vi "ReadOrSaveCases-UTEX.vi"(9 "Location":enum16{"CUMC", "SERI", "VMR", "Aline", "HSS"}(ring)=enum."SERI", 10 "New Case":T2={"Case Name"="", "Distance between\nscan lines (mm)"=0.0, "Acquistion Parameters"={"Sampling Rate"=0.0, "Ref Delay (ms)"=0.0, "rf points per line"=0, "rf lines"=0, "Dig Scale"=0.0}, "Timeout (s)"=0.0, "Sector?"=FALSE, "Filter Prams"={"low cutoff"=0, "order"=0, "high cutoff"=0}, "Scan Info"={"delay"=0.0, "pivot distance"=0.0, "sector scan angle"=0.0, "operator"="", "Scan Mode"="", "location"=""}, "UT340 Controls"={"High Pass On"=FALSE, "High Pass Filter (MHz)"=1, "Low Pass On"=FALSE, "Low Pass Filter (MHz)"=20, "PE Gain (dB)"=1, "Voltage"=100, "Pulse Width (ns)"=2.0, "Mode"=FALSE, "PC Gain (dB)"=1, "Trig Source"=FALSE, "Rep Rate (Hz)"=0, "PULSE"=FALSE}} {"UT340 Controls"."Low Pass Filter (MHz)" min=20 step=1; "UT340 Controls"."High Pass Filter (MHz)" min=1 max=20 step=1; "UT340 Controls"."Pulse Width (ns)" min=2.0 max=71.75; "UT340 Controls"."Voltage" min=100 max=250 step=2; "UT340 Controls"."PC Gain (dB)" min=0 max=63 step=1; "UT340 Controls"."PE Gain (dB)" min=-6 max=57 step=1}, 11 "Save(T)\\Read(F)":bool) -> (2 "Case List":string[](array[string]), 3 "CaseArray":T3(array[cluster]) {"UT340 Controls"."Low Pass Filter (MHz)" min=20 step=1; "UT340 Controls"."High Pass Filter (MHz)" min=1 max=20 step=1; "UT340 Controls"."Pulse Width (ns)" min=2.0 max=71.75; "UT340 Controls"."Voltage" min=100 max=250 step=2; "UT340 Controls"."PC Gain (dB)" min=0 max=63 step=1; "UT340 Controls"."PE Gain (dB)" min=-6 max=57 step=1})   [LabVIEW 2022 SP3]
uses:
  ScanningControl/Pulsers/UTEX/Controls/UTEX Controls.ctl
  ScanningControl/Digitizers/-DigitizerRoutines/Digitizer.ctl
panel:
  out "path":path
  in  "Acquistion Parameters":T4={"Sampling Rate"=250.0, "Ref Delay (ms)"=0.0, "rf points per line"=2048, "rf lines"=256, "Dig Scale"=4.0} {"Dig Scale" items=["5 V"=5.0, "2 V"=2.0, "1 V"=1.0, "500 mV"=0.5, "200 mV"=0.2, "100 mV"=0.1, "50 mV"=0.05]; "rf lines" min=1; "rf points per line" min=1; "Ref Delay (ms)" format="%.2f"}
  in  "Sector?":bool=TRUE
  in  "Filter Prams":T5={"low cutoff"=20, "order"=81, "high cutoff"=60}
  in  "Timeout (s)":dbl=0.15
  in  "Probe":T6(ring)
  in  "Scan Info":T7
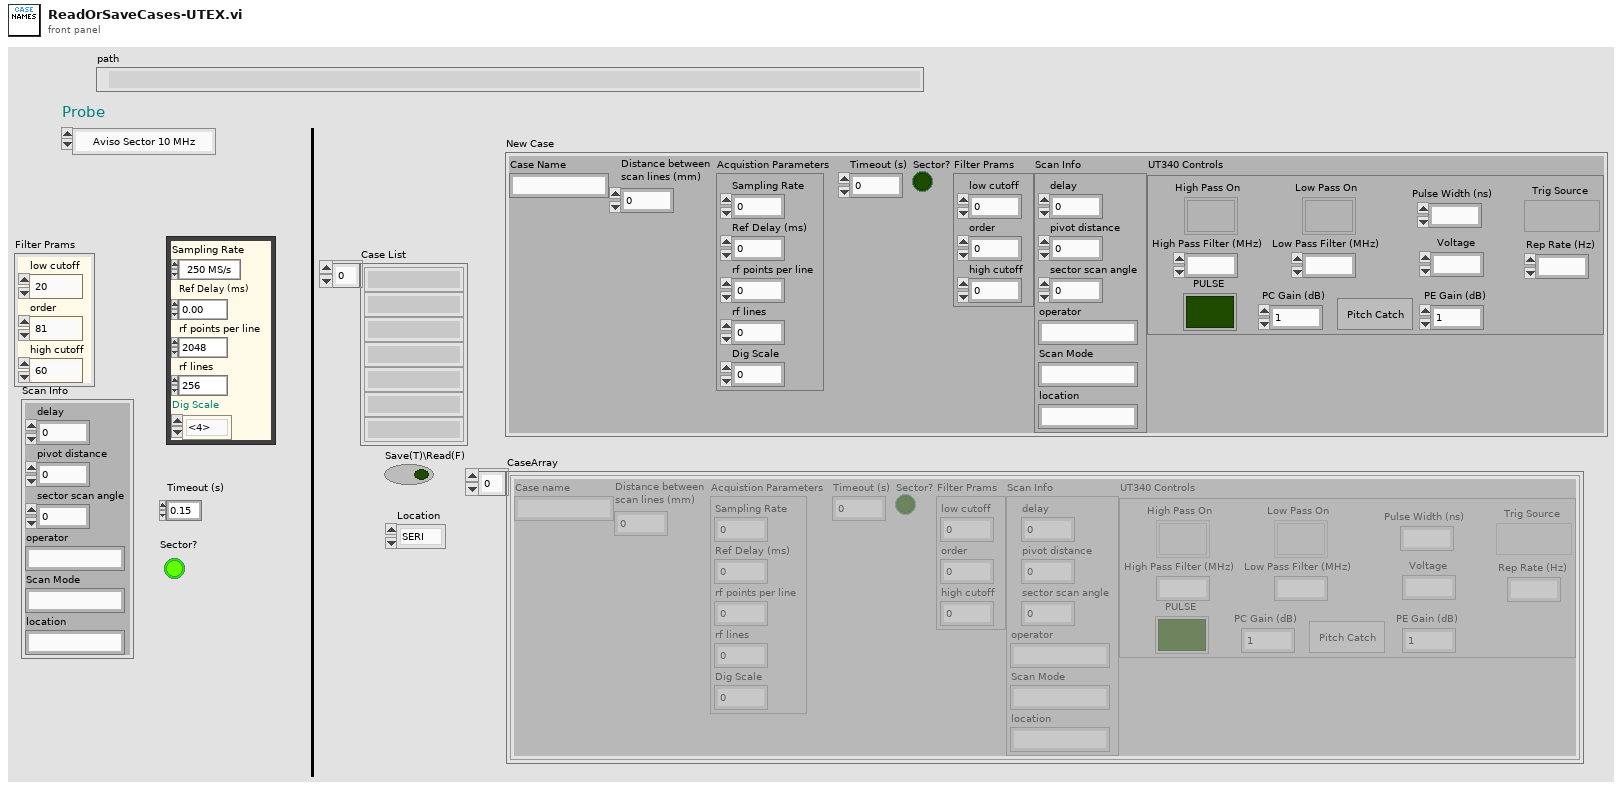
[diagram p1: front panel]
types:
  T1 = typedef "UTEX Controls.ctl" = cluster{"High Pass On":bool, "High Pass Filter (MHz)":i16, "Low Pass On":bool, "Low Pass Filter (MHz)":i16, "PE Gain (dB)":i16, "Voltage":i16, "Pulse Width (ns)":dbl, "Mode":bool, "PC Gain (dB)":i16, "Trig Source":bool, "Rep Rate (Hz)":i16, "PULSE":bool}
  T2 = cluster{"Case Name":string, "Distance between\nscan lines (mm)":sgl, "Acquistion Parameters":cluster{"Sampling Rate":dbl, "Ref Delay (ms)":dbl, "rf points per line":i32, "rf lines":i32, "Dig Scale":dbl}, "Timeout (s)":dbl, "Sector?":bool, "Filter Prams":cluster{"low cutoff":i32, "order":i32, "high cutoff":i32}, "Scan Info":cluster{"delay":sgl, "pivot distance":sgl, "sector scan angle":sgl, "operator":string, "Scan Mode":string, "location":string}, "UT340 Controls":T1}
  T3 = cluster{"Case name":string, "Distance between\nscan lines (mm)":sgl, "Acquistion Parameters":cluster{"Sampling Rate":dbl, "Ref Delay (ms)":dbl, "rf points per line":i32, "rf lines":i32, "Dig Scale":dbl}, "Timeout (s)":dbl, "Sector?":bool, "Filter Prams":cluster{"low cutoff":i32, "order":i32, "high cutoff":i32}, "Scan Info":cluster{"delay":sgl, "pivot distance":sgl, "sector scan angle":sgl, "operator":string, "Scan Mode":string, "location":string}, "UT340 Controls":T1}[]
  T4 = cluster{"Sampling Rate":dbl, "Ref Delay (ms)":dbl, "rf points per line":i32, "rf lines":i32, "Dig Scale":dbl}
  T5 = cluster{"low cutoff":i32, "order":i32, "high cutoff":i32}
  T6 = enum16{"Aviso Sector 10 MHz", "Aviso Sector 20 MHz Retina", "Aviso Sector 20 MHz", "Aviso Lin50", "UTEX 50MHz", "Custom"}
  T7 = cluster{"delay":sgl, "pivot distance":sgl, "sector scan angle":sgl, "operator":string, "Scan Mode":string, "location":string}
  T8 = typedef "Digitizer.ctl" = enum16{"Acqiris Digitizer", "NI Digitizer", "LeCroy", "GaGe", "AlazarTech", "No Digitizer", "Teledyne"}
  T9 = enum16{"open", "replace", "create", "open or create", "replace or create", "replace or create with confirmation"}
  T10 = cluster{"Case Name":string, "Distance between\nscan lines (mm)":sgl, "Acquistion Parameters":cluster{"Sampling Rate":dbl, "Ref Delay (ms)":dbl, "rf points per line":i32, "rf lines":i32, "Dig Scale":dbl}, "Timeout (s)":dbl, "Sector?":bool, "Filter Prams":cluster{"low cutoff":i32, "order":i32, "high cutoff":i32}, "Scan Info":cluster{"delay":sgl, "pivot distance":sgl, "sector scan angle":sgl, "operator":string, "Scan Mode":string, "location":string}, "UT340 Controls":T1}[]
  T11 = cluster{"Sampling Rate":dbl, "Ref Delay (ms)":dbl, "rf points per line":i32, "rf lines":i32, "Voltage Scale 1":dbl}
  T12 = cluster{"Case Name":string, "Distance between\nscan lines (mm)":sgl, "Acquistion Parameters":cluster{"Sampling Rate":dbl, "Ref Delay (ms)":dbl, "rf points per line":i32, "rf lines":i32, "Dig Scale":dbl}, "Timeout (s)":dbl, "Sector?":bool, "Filter Prams":cluster{"low cutoff":i32, "order":i32, "high cutoff":i32}, "Scan Info":cluster{"delay":sgl, "pivot distance":sgl, "sector scan angle":sgl, "operator":string, "Scan Mode":string, "location":string}}[]
  T13 = enum16{"Aviso Sector 10 MHz", "Aviso Sector 20 MHz Retina", "Aviso Sector 20 MHz", "Aviso Lin50", "Custom"}
  T14 = cluster{string, "Distance between\nscan lines (mm)":sgl, "Acquistion Parameters":cluster{"Sampling Rate":dbl, "Ref Delay (ms)":dbl, "rf points per line":i32, "rf lines":i32, "Dig Scale":dbl}, "Timeout (s)":dbl, "Sector?":bool, "Filter Prams":cluster{"low cutoff":i32, "order":i32, "high cutoff":i32}, "Scan Info":cluster{"delay":sgl, "pivot distance":sgl, "sector scan angle":sgl, "operator":string, "Scan Mode":string, "location":string}, "UT340 Controls":T1}
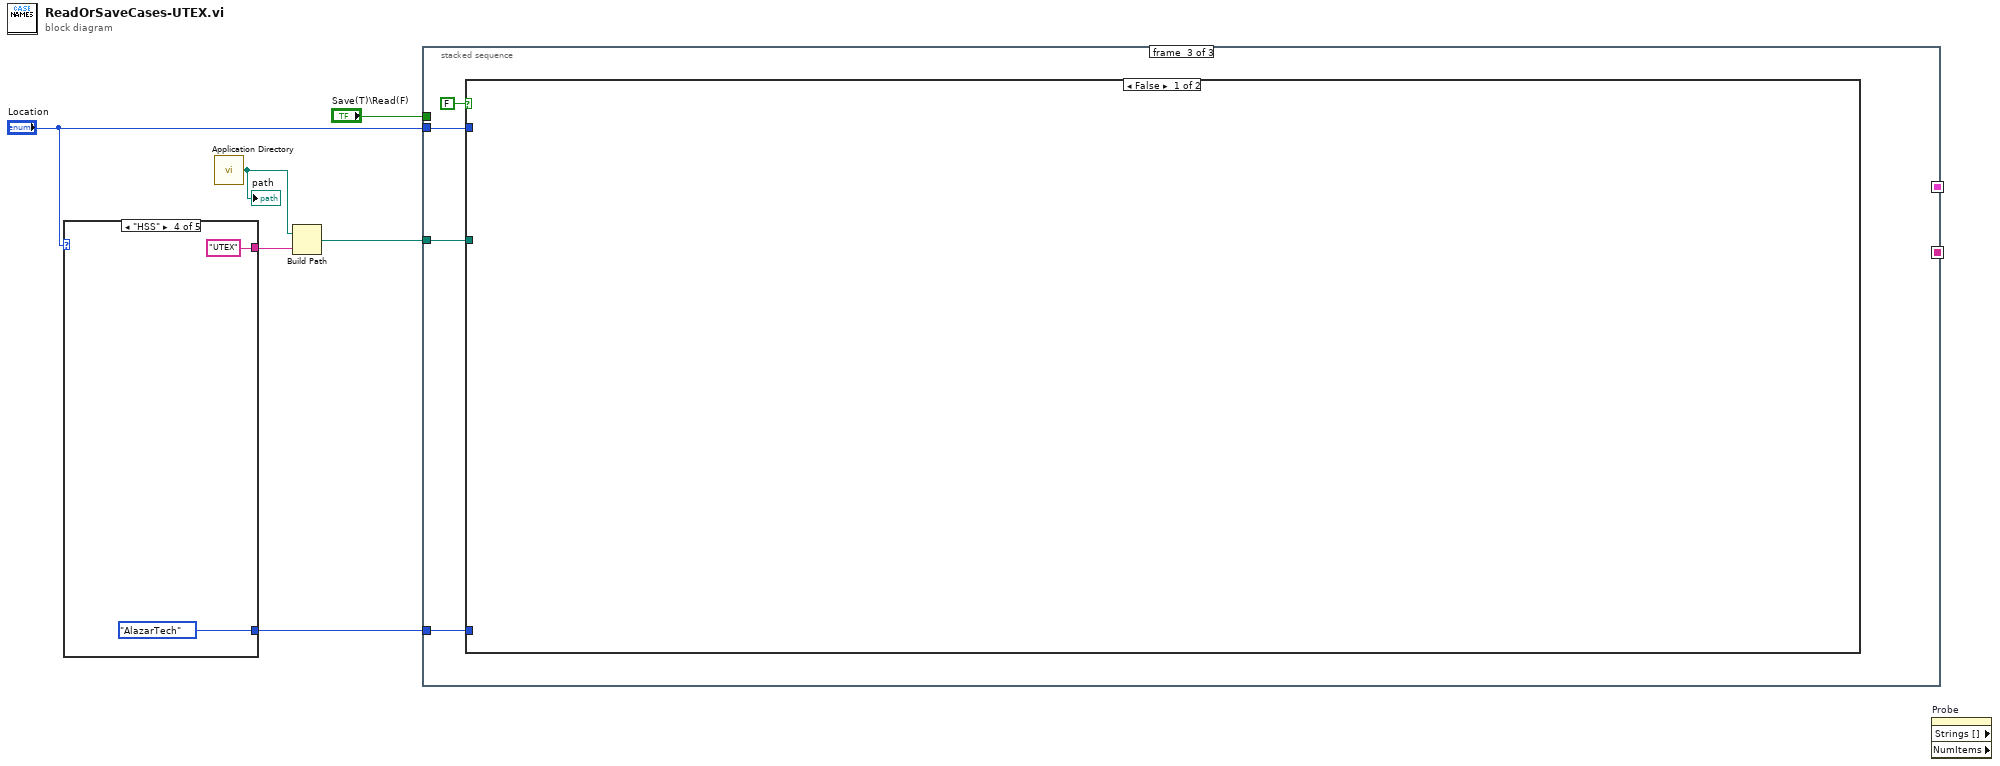
[diagram p0: block diagram]
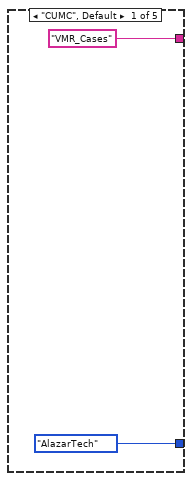
[diagram p2: hidden frame]
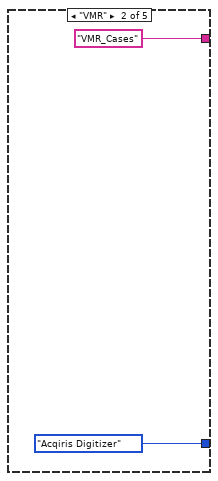
[diagram p3: hidden frame]
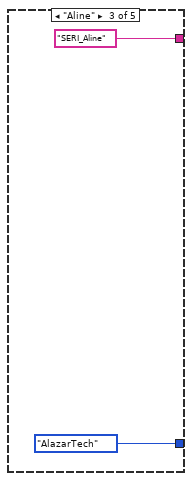
[diagram p4: hidden frame]
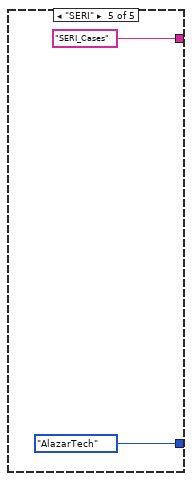
[diagram p5: hidden frame]
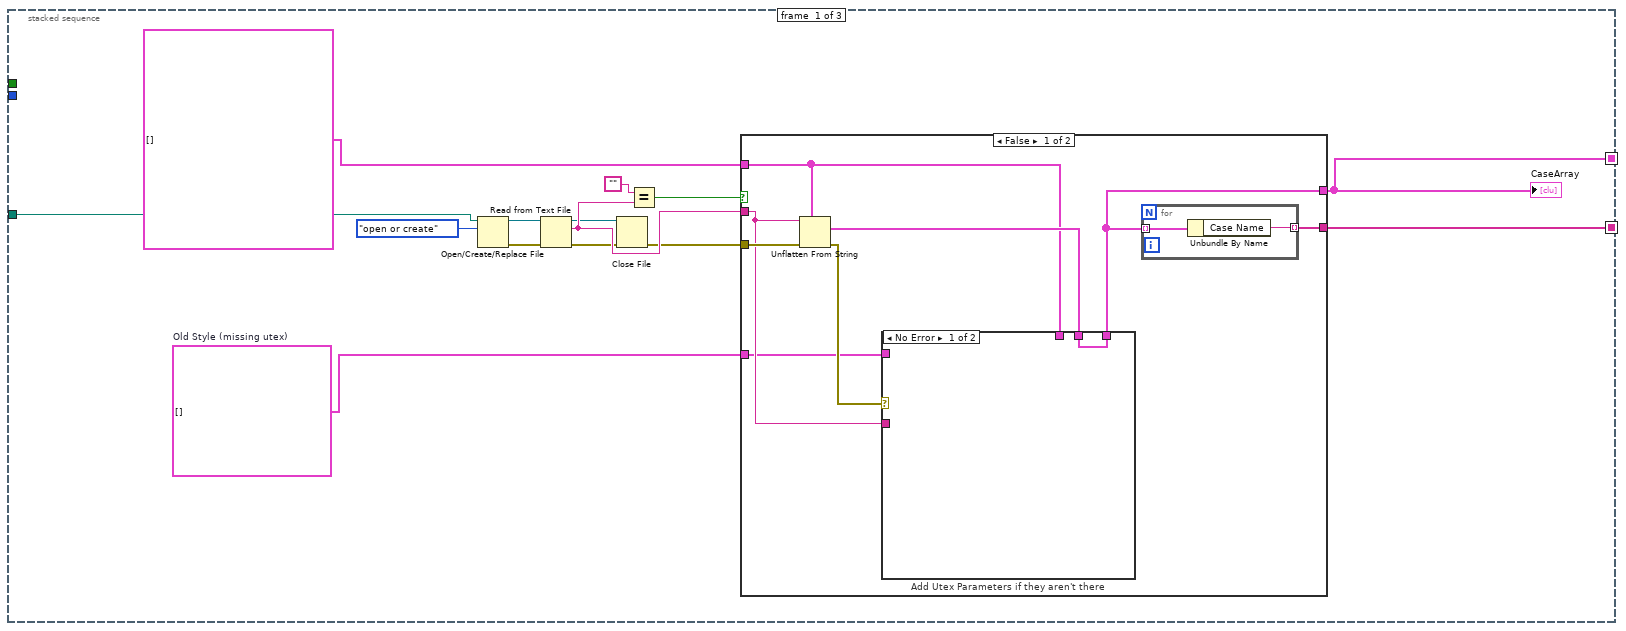
[diagram p6: hidden frame]
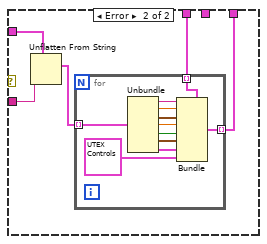
[diagram p7: hidden frame]
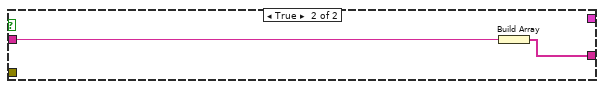
[diagram p8: hidden frame]
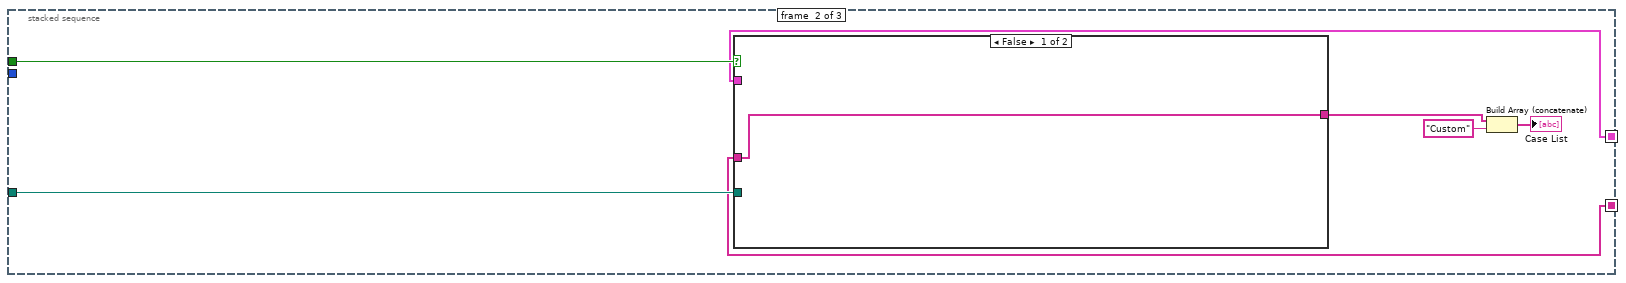
[diagram p9: hidden frame]
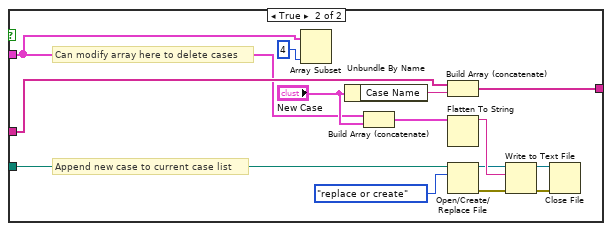
[diagram p10: hidden frame]
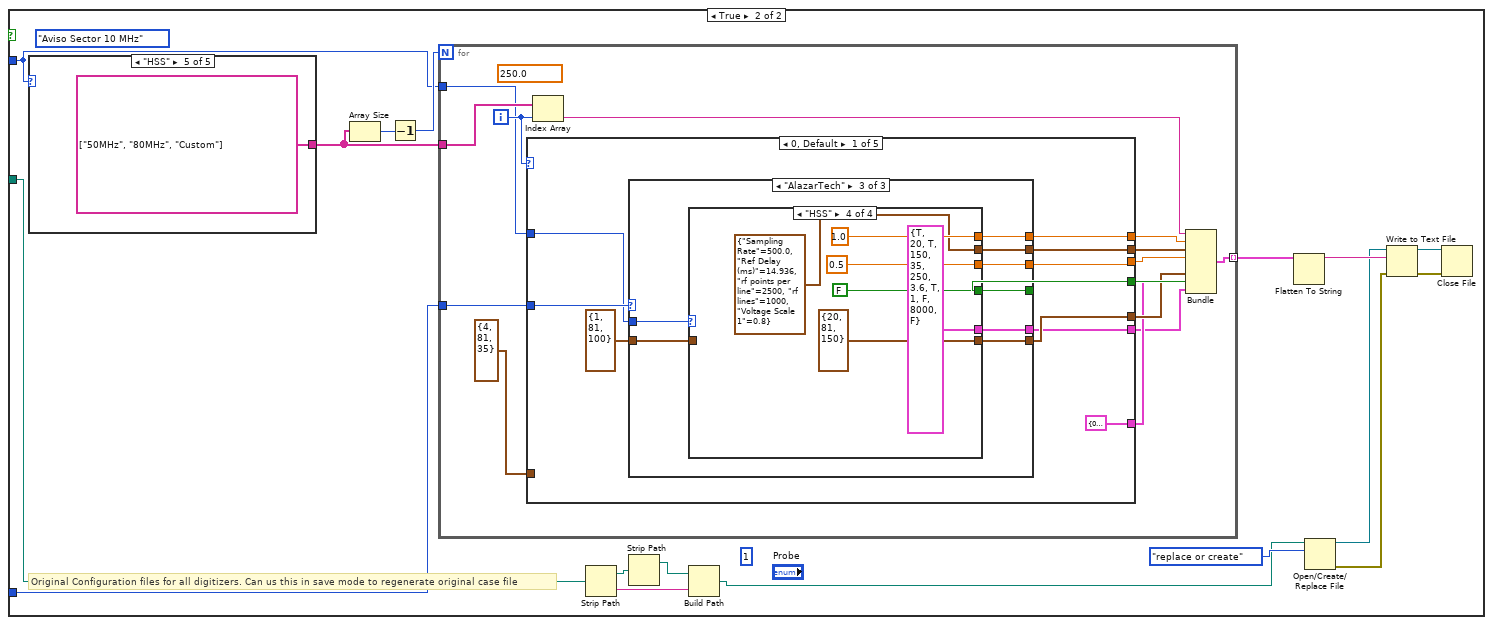
[diagram p11: hidden frame]
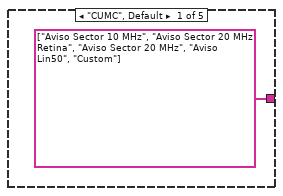
[diagram p12: hidden frame]
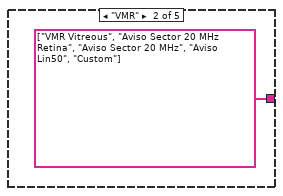
[diagram p13: hidden frame]
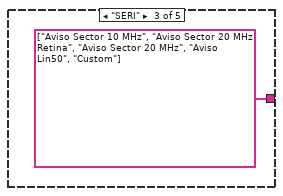
[diagram p14: hidden frame]
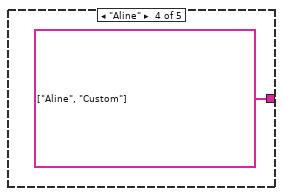
[diagram p15: hidden frame]
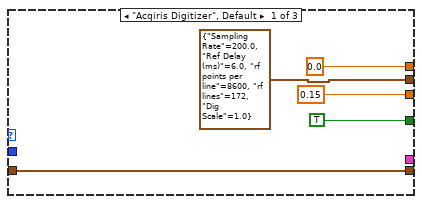
[diagram p16: hidden frame]
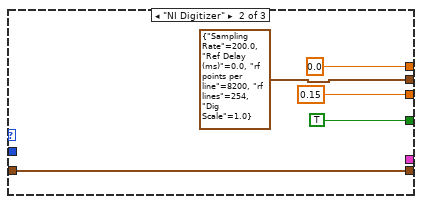
[diagram p17: hidden frame]
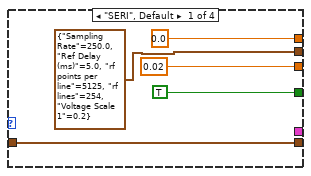
[diagram p18: hidden frame]
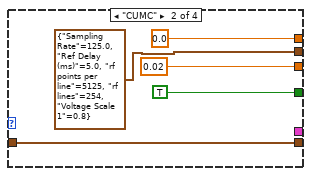
[diagram p19: hidden frame]
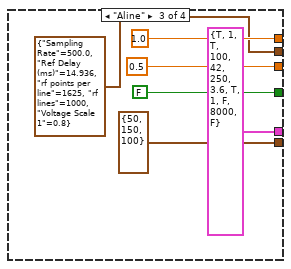
[diagram p20: hidden frame]
diagram:
  n1 = case shown="\"HSS\"" "Location" {
    tunnel: ["VMR_Cases" "VMR_Cases" "SERI_Aline" "UTEX" "SERI_Cases"] -> w4
    tunnel: [Digitizer."AlazarTech" ("Main Digitizer") Digitizer."Acqiris Digitizer" ("Main Digitizer") Digitizer."AlazarTech" ("Main Digitizer") Digitizer."AlazarTech" ("Main Digitizer") Digitizer."AlazarTech" ("Main Digitizer")] -> w1
    frame "CUMC", Default {
    }
    frame "VMR" {
    }
    frame "Aline" {
    }
    frame "HSS" {
    }
    frame "SERI" {
    }
  }
  n2 = call <vilib>:"Application Directory.vi"() -> ("Application Directory"=w3:path)
  "path" <- w3
  n3 = Build Path(base path=w3, name or relative path=w4) -> (appended path=w5:path)
  n4 = stacked-sequence {
    seq-local: [w19 _ _] -> [_ w65 _]
    seq-local: [w18 _ _] -> [_ w63 _]
    tunnel: w5 -> [w29 w64 w85]
    tunnel: "Save(T)\\Read(F)" -> [_ w66 _]
    tunnel: "Location" -> [_ _ w84]
    tunnel: w1 -> [_ _ w82]
    frame #0 {
      w17 = T12 []  # Old Style (missing utex)
      n5 = Open/Create/Replace File(file path (use dialog)=w29, operation (0:open)=T9."open or create") -> (refnum out=w28:refnum<file>, error out=w27:errorcluster)  [unwired: 4 in, 1 out]
      n6 = Read from Text File(file (use dialog)=w28, error in=w27) -> (refnum out=w20:refnum<file>, text=w24:string, error out=w22:errorcluster)  [unwired: 2 in, 1 out]
      n7 = Close File(refnum=w20, error in=w22) -> (error out=w21:errorcluster)  [unwired: 1 out]
      n8 = Equal?(x="", y=w24) -> (x = y?=w23:bool)
      n9 = case shown="False" w23 {
        tunnel: T10 [] -> [w31 _]
        tunnel: w21 -> [w38 _]
        tunnel: w24 -> [w35 w59]
        tunnel: [w37 w58] -> w18
        tunnel: [w33 _] -> w19
        tunnel: w17 -> [w34 _]
        frame False {
          n10 = Unflatten From String(type=w31, binary string=w35, error in (no error)=w38) -> (value=w32:T10, error out=w36:errorcluster)  [unwired: 2 in, 1 out]
          n11 = case "Add Utex Parameters if they aren't there" shown="No Error" w36 {
            tunnel: w35 -> [_ w44]
            tunnel: w34 -> [_ w43]
            tunnel: [w39 w41] -> w33
            tunnel: w32 -> [w39 _]
            tunnel: w31 -> [_ w40]
            frame No Error {
            }
            frame Error {
              n12 = Unflatten From String(type=w43, binary string=w44) -> (value=w42:T12)  [unwired: 3 in, 2 out]
              n13 = for {
                tunnel: w42 -> [w53] mode=indexing
                tunnel: [w55] -> w41 mode=indexing
                tunnel: w40 -> [w54] mode=indexing
                n14 = Unbundle(w53) -> ("Case Name"=w52:string, "Distance between\nscan lines (mm)"=w51:sgl, "Acquistion Parameters"=w50:T4, "Timeout (s)"=w49:dbl, "Sector?"=w48:bool, "Filter Prams"=w47:T5, "Scan Info"=w46:T7)
                n15 = Bundle(cluster=w54, "Case Name"=w52, "Distance between\nscan lines (mm)"=w51, "Acquistion Parameters"=w50, "Timeout (s)"=w49, "Sector?"=w48, "Filter Prams"=w47, "Scan Info"=w46, "UT340 Controls"=T1 {"High Pass On"=FALSE, "High Pass Filter (MHz)"=1, "Low Pass On"=FALSE, "Low Pass Filter (MHz)"=20, "PE Gain (dB)"=1, "Voltage"=100, "Pulse Width (ns)"=2.0, "Mode"=FALSE, "PC Gain (dB)"=1, "Trig Source"=FALSE, "Rep Rate (Hz)"=0, "PULSE"=FALSE}) -> (w55:T2)
              }
            }
          }
          n16 = for {
            tunnel: w33 -> [w57] mode=indexing
            tunnel: [w56] -> w37 mode=indexing
            n17 = Unbundle By Name(w57) -> ("Case Name"=w56:string)
          }
        }
        frame True {
          n18 = Build Array(w59) -> (w58:string[])
        }
      }
      "CaseArray" <- w19
    }
    frame #1 {
      n19 = case shown="False" w66 {
        tunnel: w65 -> [_ w70]
        tunnel: w64 -> [_ w75]
        tunnel: w63 -> [w67 w73]
        tunnel: [w67 w71] -> w62
        frame False {
        }
        frame True {
          # "Can modify array here to delete cases"
          # "Append new case to current case list"
          n20 = Array Subset(array=w70, length=4) -> ()  [unwired: 1 in, 1 out]
          n21 = Unbundle By Name("New Case") -> ("Case Name"=w72:string)
          n22 = Build Array (concatenate)(w70, "New Case") -> (w68:T10)
          n23 = Build Array (concatenate)(w73, w72) -> (w71:string[])
          n24 = Flatten To String(anything=w68) -> (data string=w81:string)  [unwired: 3 in, 2 out]
          n25 = Open/Create/Replace File(file path (use dialog)=w75, operation (0:open)=T9."replace or create") -> (refnum out=w77:refnum<file>, error out=w78:errorcluster)  [unwired: 4 in, 1 out]
          n26 = Write to Text File(file (use dialog)=w77, text=w81, error in=w78) -> (refnum out=w80:refnum<file>, error out=w79:errorcluster)  [unwired: 1 in, 1 out]
          n27 = Close File(refnum=w80, error in=w79) -> ()  [unwired: 2 out]
        }
      }
      n28 = Build Array (concatenate)(w62, "Custom" ("Case Name")) -> (→"Case List":string[])
    }
    frame #2 {
      n29 = case shown="False" FALSE {
        tunnel: w85 -> [_ w90]
        tunnel: w84 -> [_ w94]
        tunnel: w82 -> [_ w91]
        frame False {
        }
        frame True {
          (unwired) 1
          (unwired) T13."Aviso Sector 10 MHz" ("Probe")
          # "Original Configuration files for all digitizers. Can us this in save mode to regenerate original case file"
          n30 = case shown="\"HSS\"" w94 {
            tunnel: [string[] ["Aviso Sector 10 MHz", "Aviso Sector 20 MHz Retina", "Aviso Sector 20 MHz", "Aviso Lin50", "Custom"] ("Strings []") string[] ["VMR Vitreous", "Aviso Sector 20 MHz Retina", "Aviso Sector 20 MHz", "Aviso Lin50", "Custom"] ("Strings []") string[] ["Aviso Sector 10 MHz", "Aviso Sector 20 MHz Retina", "Aviso Sector 20 MHz", "Aviso Lin50", "Custom"] ("Strings []") string[] ["Aline", "Custom"] ("Strings []") string[] ["50MHz", "80MHz", "Custom"] ("Strings []")] -> w93
            frame "CUMC", Default {
            }
            frame "VMR" {
            }
            frame "SERI" {
            }
            frame "Aline" {
            }
            frame "HSS" {
            }
          }
          n31 = Array Size(array=w93) -> (size(s)=w92:i32)
          n32 = Decrement(x=w92) -> (x-1=w95:i32)
          n33 = for {
            N: w95 -> [_]
            tunnel: w93 -> [w112]
            tunnel: [w114] -> w100 mode=indexing
            tunnel: w94 -> [w111]
            tunnel: w91 -> [w110]
            i -> [w113]
            (unwired) 250.0 ("Sampling Rate")
            n34 = case shown="0, Default" w113 {
              tunnel: [w125 sgl 0.0 sgl 0.0 sgl 50.0 sgl 0.0 ("Distance between\nscan lines (mm)")] -> w121
              tunnel: [w131 w180 w221 w239 "Acquistion Parameters"] -> w120
              tunnel: [w123 w173 T5 {"low cutoff"=4, "order"=81, "high cutoff"=35} ("Filter Prams") T5 {"low cutoff"=20, "order"=81, "high cutoff"=60} ("Filter Prams") "Filter Prams"] -> w117
              tunnel: [T7 {"delay"=0.0, "pivot distance"=9.0, "sector scan angle"=50.0, "operator"="", "Scan Mode"="", "location"=""} ("Scan Info") T7 {"delay"=0.0, "pivot distance"=9.0, "sector scan angle"=50.0, "operator"="", "Scan Mode"="", "location"=""} ("Scan Info") T7 {"delay"=0.0, "pivot distance"=9.0, "sector scan angle"=50.0, "operator"="", "Scan Mode"="", "location"=""} ("Scan Info") T7 {"delay"=0.0, "pivot distance"=0.0, "sector scan angle"=0.0, "operator"="", "Scan Mode"="", "location"=""} ("Scan Info") "Scan Info"] -> w116
              tunnel: w110 -> [w129 w178 w218 w240 _]
              tunnel: [w128 w177 w217 w238 "Timeout (s)"] -> w119
              tunnel: [w126 w175 TRUE FALSE "Sector?"] -> w118
              tunnel: w111 -> [w127 w176 w215 w236 _]
              tunnel: [w122 w174 _ _ _] -> w109
              tunnel: T5 {"low cutoff"=4, "order"=81, "high cutoff"=35} ("Filter Prams") -> [_ w172 _ _ _]
              frame 0, Default {
                n35 = case shown="\"AlazarTech\"" w129 {
                  tunnel: [T4 {"Sampling Rate"=200.0, "Ref Delay (ms)"=6.0, "rf points per line"=8600, "rf lines"=172, "Dig Scale"=1.0} ("Acquistion Parameters") T4 {"Sampling Rate"=200.0, "Ref Delay (ms)"=0.0, "rf points per line"=8200, "rf lines"=254, "Dig Scale"=1.0} ("RF data Sampling") w149] -> w131
                  tunnel: [0.15 ("Timeout (s)") 0.15 ("Timeout (s)") w148] -> w128
                  tunnel: w127 -> [_ _ w147]
                  tunnel: [TRUE TRUE w146] -> w126
                  tunnel: [sgl 0.0 sgl 0.0 w145] -> w125
                  tunnel: [w132 w137 w144] -> w123
                  tunnel: T5 {"low cutoff"=1, "order"=81, "high cutoff"=100} ("Filter Prams") -> [w132 w137 w143]
                  tunnel: [_ _ w142] -> w122
                  frame "Acqiris Digitizer", Default {
                  }
                  frame "NI Digitizer" {
                  }
                  frame "AlazarTech" {
                    n36 = case shown="\"HSS\"" w147 {
                      tunnel: [T11 {"Sampling Rate"=250.0, "Ref Delay (ms)"=5.0, "rf points per line"=5125, "rf lines"=254, "Voltage Scale 1"=0.2} ("RF data Sampling") T11 {"Sampling Rate"=125.0, "Ref Delay (ms)"=5.0, "rf points per line"=5125, "rf lines"=254, "Voltage Scale 1"=0.8} ("RF data Sampling") T11 {"Sampling Rate"=500.0, "Ref Delay (ms)"=14.936, "rf points per line"=1625, "rf lines"=1000, "Voltage Scale 1"=0.8} ("RF data Sampling") T11 {"Sampling Rate"=500.0, "Ref Delay (ms)"=14.936, "rf points per line"=2500, "rf lines"=1000, "Voltage Scale 1"=0.8} ("RF data Sampling")] -> w149
                      tunnel: [0.02 ("Timeout (s)") 0.02 ("Timeout (s)") 0.5 ("Timeout (s)") 0.5 ("Timeout (s)")] -> w148
                      tunnel: [TRUE TRUE FALSE FALSE] -> w146
                      tunnel: [sgl 0.0 sgl 0.0 sgl 1.0 sgl 1.0] -> w145
                      tunnel: [w150 w155 T5 {"low cutoff"=50, "order"=150, "high cutoff"=100} ("Filter Prams") T5 {"low cutoff"=20, "order"=81, "high cutoff"=150} ("Filter Prams")] -> w144
                      tunnel: w143 -> [w150 w155 _ _]
                      tunnel: [_ _ T1 {"High Pass On"=TRUE, "High Pass Filter (MHz)"=1, "Low Pass On"=TRUE, "Low Pass Filter (MHz)"=100, "PE Gain (dB)"=42, "Voltage"=250, "Pulse Width (ns)"=3.6, "Mode"=TRUE, "PC Gain (dB)"=1, "Trig Source"=FALSE, "Rep Rate (Hz)"=8000, "PULSE"=FALSE} ("UT340 Controls") T1 {"High Pass On"=TRUE, "High Pass Filter (MHz)"=20, "Low Pass On"=TRUE, "Low Pass Filter (MHz)"=150, "PE Gain (dB)"=35, "Voltage"=250, "Pulse Width (ns)"=3.6, "Mode"=TRUE, "PC Gain (dB)"=1, "Trig Source"=FALSE, "Rep Rate (Hz)"=8000, "PULSE"=FALSE} ("UT340 Controls")] -> w142
                      frame "SERI", Default {
                      }
                      frame "CUMC" {
                      }
                      frame "Aline" {
                      }
                      frame "HSS" {
                      }
                    }
                  }
                }
              }
              frame 1 {
                n37 = case shown="\"AlazarTech\"" w178 {
                  tunnel: [T4 {"Sampling Rate"=200.0, "Ref Delay (ms)"=30.0, "rf points per line"=3000, "rf lines"=169, "Dig Scale"=0.05} ("Acquistion Parameters") T4 {"Sampling Rate"=200.0, "Ref Delay (ms)"=0.0, "rf points per line"=8200, "rf lines"=254, "Dig Scale"=1.0} ("RF data Sampling") w196] -> w180
                  tunnel: [0.08 ("Timeout (s)") 0.15 ("Timeout (s)") w195] -> w177
                  tunnel: w176 -> [_ _ w194]
                  tunnel: [TRUE TRUE w193] -> w175
                  tunnel: [_ _ w192] -> w174
                  tunnel: [w182 w186 w190] -> w173
                  tunnel: w172 -> [w182 w186 w191]
                  frame "Acqiris Digitizer", Default {
                  }
                  frame "NI Digitizer" {
                  }
                  frame "AlazarTech" {
                    n38 = case shown="\"HSS\"" w194 {
                      tunnel: [T11 {"Sampling Rate"=250.0, "Ref Delay (ms)"=5.0, "rf points per line"=5125, "rf lines"=254, "Voltage Scale 1"=0.2} ("RF data Sampling") T11 {"Sampling Rate"=125.0, "Ref Delay (ms)"=30.0, "rf points per line"=3000, "rf lines"=254, "Voltage Scale 1"=0.8} ("RF data Sampling") T11 {"Sampling Rate"=500.0, "Ref Delay (ms)"=5.0, "rf points per line"=1000, "rf lines"=1000, "Voltage Scale 1"=0.8} ("RF data Sampling") T11 {"Sampling Rate"=500.0, "Ref Delay (ms)"=0.0, "rf points per line"=2500, "rf lines"=1000, "Voltage Scale 1"=0.8} ("RF data Sampling")] -> w196
                      tunnel: [0.02 ("Timeout (s)") 0.02 ("Timeout (s)") 0.02 ("Timeout (s)") 0.02 ("Timeout (s)")] -> w195
                      tunnel: [TRUE TRUE FALSE FALSE] -> w193
                      tunnel: [_ _ T1 {"High Pass On"=TRUE, "High Pass Filter (MHz)"=10, "Low Pass On"=TRUE, "Low Pass Filter (MHz)"=100, "PE Gain (dB)"=42, "Voltage"=100, "Pulse Width (ns)"=2.0, "Mode"=TRUE, "PC Gain (dB)"=1, "Trig Source"=FALSE, "Rep Rate (Hz)"=1000, "PULSE"=TRUE} ("UT340 Controls") T1 {"High Pass On"=TRUE, "High Pass Filter (MHz)"=20, "Low Pass On"=TRUE, "Low Pass Filter (MHz)"=150, "PE Gain (dB)"=35, "Voltage"=250, "Pulse Width (ns)"=2.0, "Mode"=TRUE, "PC Gain (dB)"=1, "Trig Source"=FALSE, "Rep Rate (Hz)"=8000, "PULSE"=FALSE} ("UT340 Controls")] -> w192
                      tunnel: [w197 w201 w205 T5 {"low cutoff"=20, "order"=81, "high cutoff"=150} ("Filter Prams")] -> w190
                      tunnel: w191 -> [w197 w201 w205 _]
                      frame "SERI", Default {
                      }
                      frame "CUMC" {
                      }
                      frame "Aline" {
                      }
                      frame "HSS" {
                      }
                    }
                  }
                }
              }
              frame 2 {
                n39 = case shown="\"AlazarTech\"" w218 {
                  tunnel: [T4 {"Sampling Rate"=200.0, "Ref Delay (ms)"=5.0, "rf points per line"=8000, "rf lines"=168, "Dig Scale"=0.05} ("Acquistion Parameters") T4 {"Sampling Rate"=250.0, "Ref Delay (ms)"=5.0, "rf points per line"=10250, "rf lines"=254, "Dig Scale"=1.0} ("RF data Sampling") w229] -> w221
                  tunnel: [0.08 ("Timeout (s)") 0.15 ("Timeout (s)") w228] -> w217
                  tunnel: w215 -> [_ _ w227]
                  frame "Acqiris Digitizer", Default {
                  }
                  frame "NI Digitizer" {
                  }
                  frame "AlazarTech" {
                    n40 = case shown="\"HSS\"" w227 {
                      tunnel: [T11 {"Sampling Rate"=250.0, "Ref Delay (ms)"=5.0, "rf points per line"=5125, "rf lines"=254, "Voltage Scale 1"=0.2} ("RF data Sampling") T11 {"Sampling Rate"=500.0, "Ref Delay (ms)"=2.468, "rf points per line"=650, "rf lines"=254, "Voltage Scale 1"=0.2} ("RF data Sampling") T11 {"Sampling Rate"=125.0, "Ref Delay (ms)"=5.0, "rf points per line"=5125, "rf lines"=254, "Voltage Scale 1"=0.4} ("RF data Sampling")] -> w229
                      tunnel: [0.02 ("Timeout (s)") 0.02 ("Timeout (s)") 0.02 ("Timeout (s)")] -> w228
                      frame "SERI", Default {
                      }
                      frame "HSS" {
                      }
                      frame "CUMC" {
                      }
                    }
                  }
                }
              }
              frame 3 {
                n41 = case shown="\"NI Digitizer\"" w240 {
                  tunnel: [T4 {"Sampling Rate"=400.0, "Ref Delay (ms)"=5.4, "rf points per line"=8000, "rf lines"=254, "Dig Scale"=0.5} ("Acquistion Parameters") T4 {"Sampling Rate"=250.0, "Ref Delay (ms)"=5.4, "rf points per line"=5000, "rf lines"=254, "Dig Scale"=0.4} ("RF data Sampling") w250] -> w239
                  tunnel: [0.08 ("Timeout (s)") 0.15 ("Timeout (s)") w249] -> w238
                  tunnel: w236 -> [_ _ w248]
                  frame "Acqiris Digitizer", Default {
                  }
                  frame "NI Digitizer" {
                  }
                  frame "AlazarTech" {
                    n42 = case shown="\"SERI\", Default" w248 {
                      tunnel: [T11 {"Sampling Rate"=250.0, "Ref Delay (ms)"=5.0, "rf points per line"=5125, "rf lines"=254, "Voltage Scale 1"=0.2} ("RF data Sampling") T11 {"Sampling Rate"=125.0, "Ref Delay (ms)"=5.4, "rf points per line"=2500, "rf lines"=254, "Voltage Scale 1"=0.8} ("RF data Sampling")] -> w250
                      tunnel: [0.02 ("Timeout (s)") 0.02 ("Timeout (s)")] -> w249
                      frame "SERI", Default {
                      }
                      frame "CUMC" {
                      }
                    }
                  }
                }
              }
              frame 4 {
              }
            }
            n43 = Index Array(array=w112, index=w113) -> (element=w115:string)
            n44 = Bundle(w115, "Distance between\nscan lines (mm)"=w121, "Acquistion Parameters"=w120, "Timeout (s)"=w119, "Sector?"=w118, "Filter Prams"=w117, "Scan Info"=w116, "UT340 Controls"=w109) -> (w114:T14)  [unwired: 1 in]
          }
          n45 = Strip Path(path=w90) -> (stripped path=w89:path, name=w87:string)
          n46 = Strip Path(path=w89) -> (stripped path=w88:path)  [unwired: 1 out]
          n47 = Build Path(base path=w88, name or relative path=w87) -> (appended path=w86:path)
          n48 = Flatten To String(anything=w100) -> (data string=w102:string)  [unwired: 3 in, 2 out]
          n49 = Open/Create/Replace File(file path (use dialog)=w86, operation (0:open)=T9."replace or create") -> (refnum out=w97:refnum<file>, error out=w98:errorcluster)  [unwired: 4 in, 1 out]
          n50 = Write to Text File(file (use dialog)=w97, text=w102, error in=w98) -> (refnum out=w101:refnum<file>, error out=w99:errorcluster)  [unwired: 1 in, 1 out]
          n51 = Close File(refnum=w101, error in=w99) -> ()  [unwired: 2 out]
        }
      }
    }
  }
  n52 = property on="Probe" class="Enum (strict)" props=["Strings []", "NumItems"]() -> ()  [unwired: 2 in, 4 out]
